vi "Write RequestHeaderContentFirst.vi"(8 "error in (no error)":errorcluster, 10 "RequestHeaderContentFirst":bool, 11 "LabVIEWHTTPClient_NET in":refnum<class "HttpClient_NET.lvclass">) -> (0 "error out":errorcluster, 3 "LabVIEWHTTPClient_NET out":refnum<class "HttpClient_NET.lvclass">)   [LabVIEW 2018, in "HttpClient_NET.lvlib" / "HttpClient_NET.lvclass"]
doc: "<b> </b> <b> </b>\nHttpClient_NET\nJustin Young - Viviota\nCopyright (c) 2021\nLicense: BSD"
uses:
  HttpClient_NET.lvclass
  HttpClient_NET.lvclass/HttpClient_NET.ctl
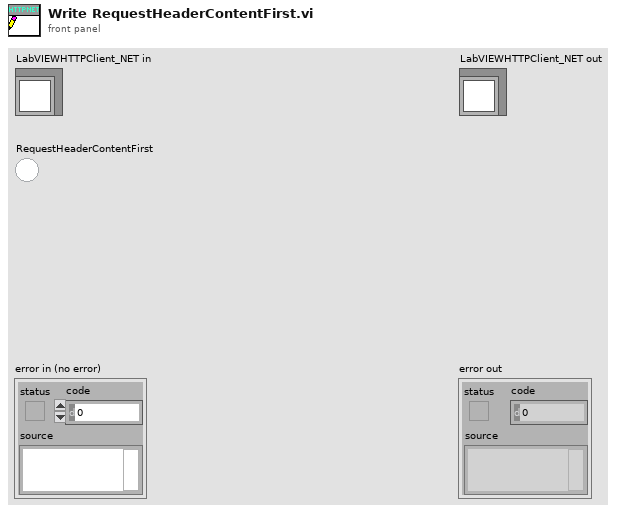
[diagram p1: front panel]
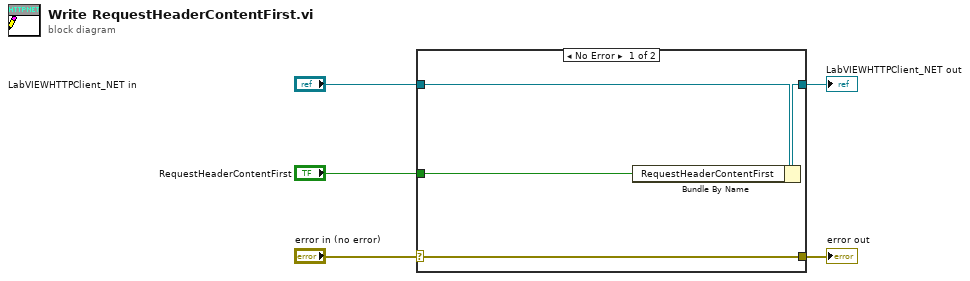
[diagram p0: block diagram]
diagram:
  n1 = case shown="No Error" "error in (no error)" {
    selector: "error in (no error)" -> [w9 w10]
    tunnel: [w9 w10] -> w4
    tunnel: [w7 w11] -> w2
    tunnel: "LabVIEWHTTPClient_NET in" -> [w8 w11]
    tunnel: "RequestHeaderContentFirst" -> [w6 _]
    frame No Error {
      n2 = Bundle By Name(cluster=w8, "RequestHeaderContentFirst"=w6) -> (w7:refnum<class "HttpClient_NET.lvclass">)
    }
    frame Error {
    }
  }
  "error out" <- w4
  "LabVIEWHTTPClient_NET out" <- w2
